vi "Close MeasurementLink Session.vi"(8 "error in (no error)":errorcluster, 9 "initialize and close session behavior":T1, 10 "session in":variant, 11 "instrument in":refnum<class "Fake Session Factory.lvclass">) -> (0 "error out":errorcluster)   [LabVIEW 2020, in "MeasurementServerTests.lvlib" / "Fake Session Factory.lvclass"]
uses:
  Fake Session Factory.lvclass
  Runtime/MeasurementLink Instrument/ISession Factory/Initialize and Close Session Behavior.ctl
  Call Recorder Action.ctl
  Runtime/MeasurementLink Instrument/ISession Factory/ISession Factory.lvclass
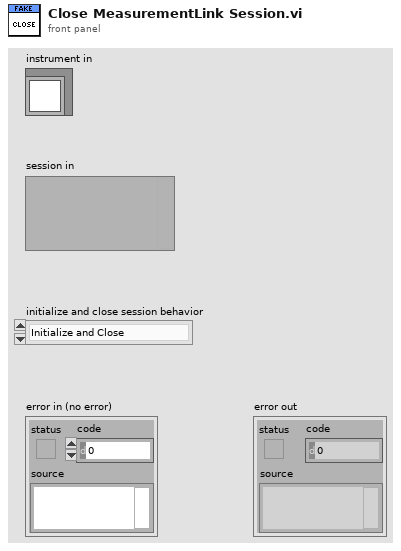
[diagram p1: front panel]
types:
  T1 = typedef "MeasurementLink Instrument.lvlib/ISession Factory.lvclass/Initialize and Close Session Behavior.ctl" = enum16{"Initialize and Close", "Attach and Detach", "Initialize and Detach", "Attach and Close"}
  T2 = typedef "MeasurementServerTests.lvlib/Fake Session Factory.lvclass/Call Recorder Action.ctl" = enum16{"Initialize", "Read Values", "Record Initialize-Initialize", "Record Initialize-Attach", "Record Close-Close", "Record Close-Detach"}
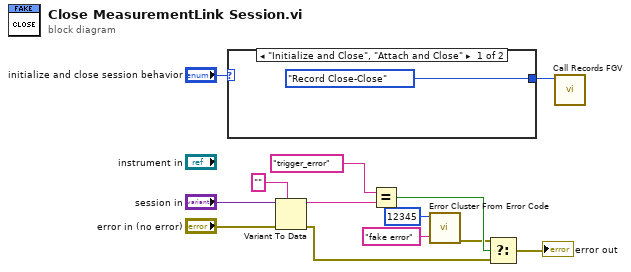
[diagram p0: block diagram]
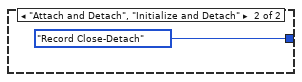
[diagram p2: hidden frame]
diagram:
  n1 = case shown="\"Initialize and Close\", \"Attach and Close\"" "initialize and close session behavior" {
    tunnel: [Call_Recorder_Action."Record Close-Close" ("Call Recorder Action") Call_Recorder_Action."Record Close-Detach" ("Call Recorder Action")] -> w12
    frame "Initialize and Close", "Attach and Close" {
    }
    frame "Attach and Detach", "Initialize and Detach" {
    }
  }
  n2 = Variant To Data(error in="error in (no error)", type="", Variant="session in") -> (data=w4:string, error out=w2:errorcluster)
  n3 = Equal?(x="trigger_error" ("y"), y=w4) -> (x = y?=w6:bool)
  n4 = call <vilib>:"Error Cluster From Error Code.vi"("error message (\"\")"="fake error" ("error message (\"\")"), "error code (0)"=12345) -> ("error out"=w5:errorcluster)  [unwired: 7 in]
  n5 = Select(t=w5, s=w6, f=w2) -> (s? t:f=→"error out":errorcluster)
  n6 = call "Call Records FGV.vi"("Call Recorder Action"=w12) -> ()  [unwired: 7 in, 4 out]
